vi "Galil Terminal.vi"(6 "Disable?":bool, 7 "Command Input":string, 10 "Galil Error In":errorcluster, 11 "reference out 2":refnum<k7>) -> (2 "Galil Error Out":errorcluster, 3 "reference out 3":refnum<k7>, 5 "Command Output":string)   [LabVIEW 2011]
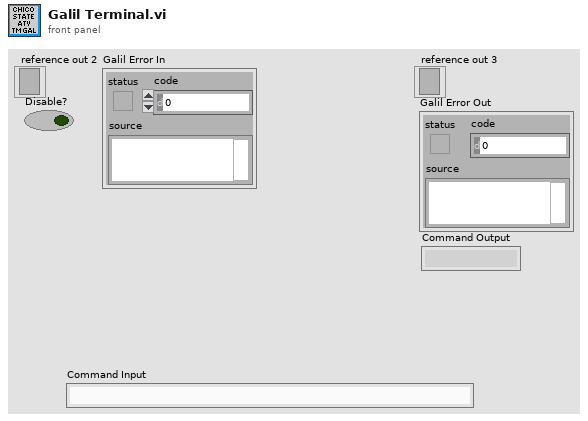
[diagram p1: front panel]
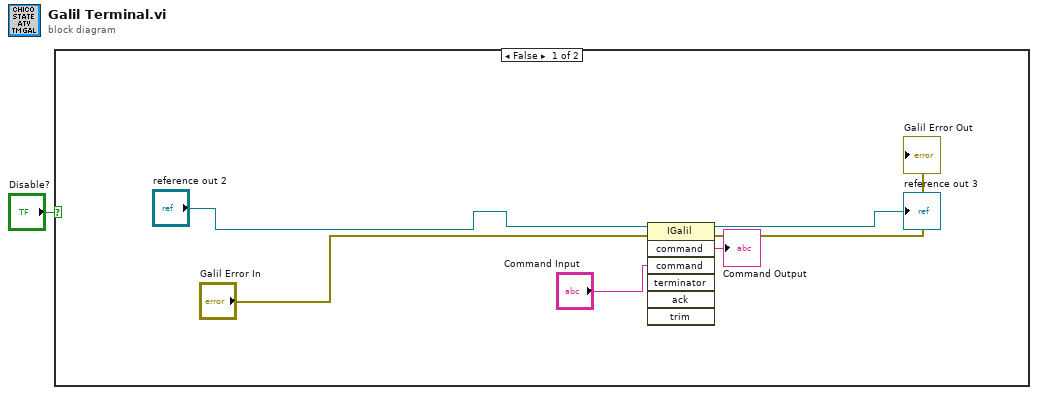
[diagram p0: block diagram]
diagram:
  n1 = case shown="False" "Disable?" {
    frame False {
      n2 = invoke class="IGalil" method="command"(reference="reference out 2", error in="Galil Error In", "command"="Command Input") -> (reference out=→"reference out 3":refnum<k7>, error out=→"Galil Error Out":errorcluster, "command"=→"Command Output":string)  [unwired: 4 in, 4 out]
    }
    frame True {
    }
  }
